vi "2DScan.vi"() -> ()   [LabVIEW 2014]
uses:
  <vilib>/vision/driver/IMAQdx.llb/IMAQdx Acquisition Mode.ctl
  <vilib>/vision/driver/IMAQdx.llb/IMAQdx Buffer Number Mode.ctl
  <vilib>/vision/driver/NI_Vision_Acquisition_Software.lvlib
panel:
  in  "Distance(V)":dbl
  in  "Boolean":bool
  out "RealPositionX":dbl
  out "Processed Frames/s":dbl
  in  "Step(V) Y":dbl=0.1
  out "RealPositionY":dbl
  in  "Step(V) X":dbl=0.1
  in  "pfVoltage in 2":sgl
  in  "pfVoltage in":sgl
  in  "Camera Name":refnum<k21>="cam0" caption="IMAQdx Session"
  in  "Stop":bool
  out "Image":T1(plugin-control)
  out "Buffer Number":u32
  out "error out":errorcluster
  in  "MG17Piezo X":refnum<k7>(container)
  in  "MG17Piezo Y":refnum<k7>(container)
  in  "MG17Piezo Z":refnum<k7>(container)
  # "2DScan"
  # "Randomic"
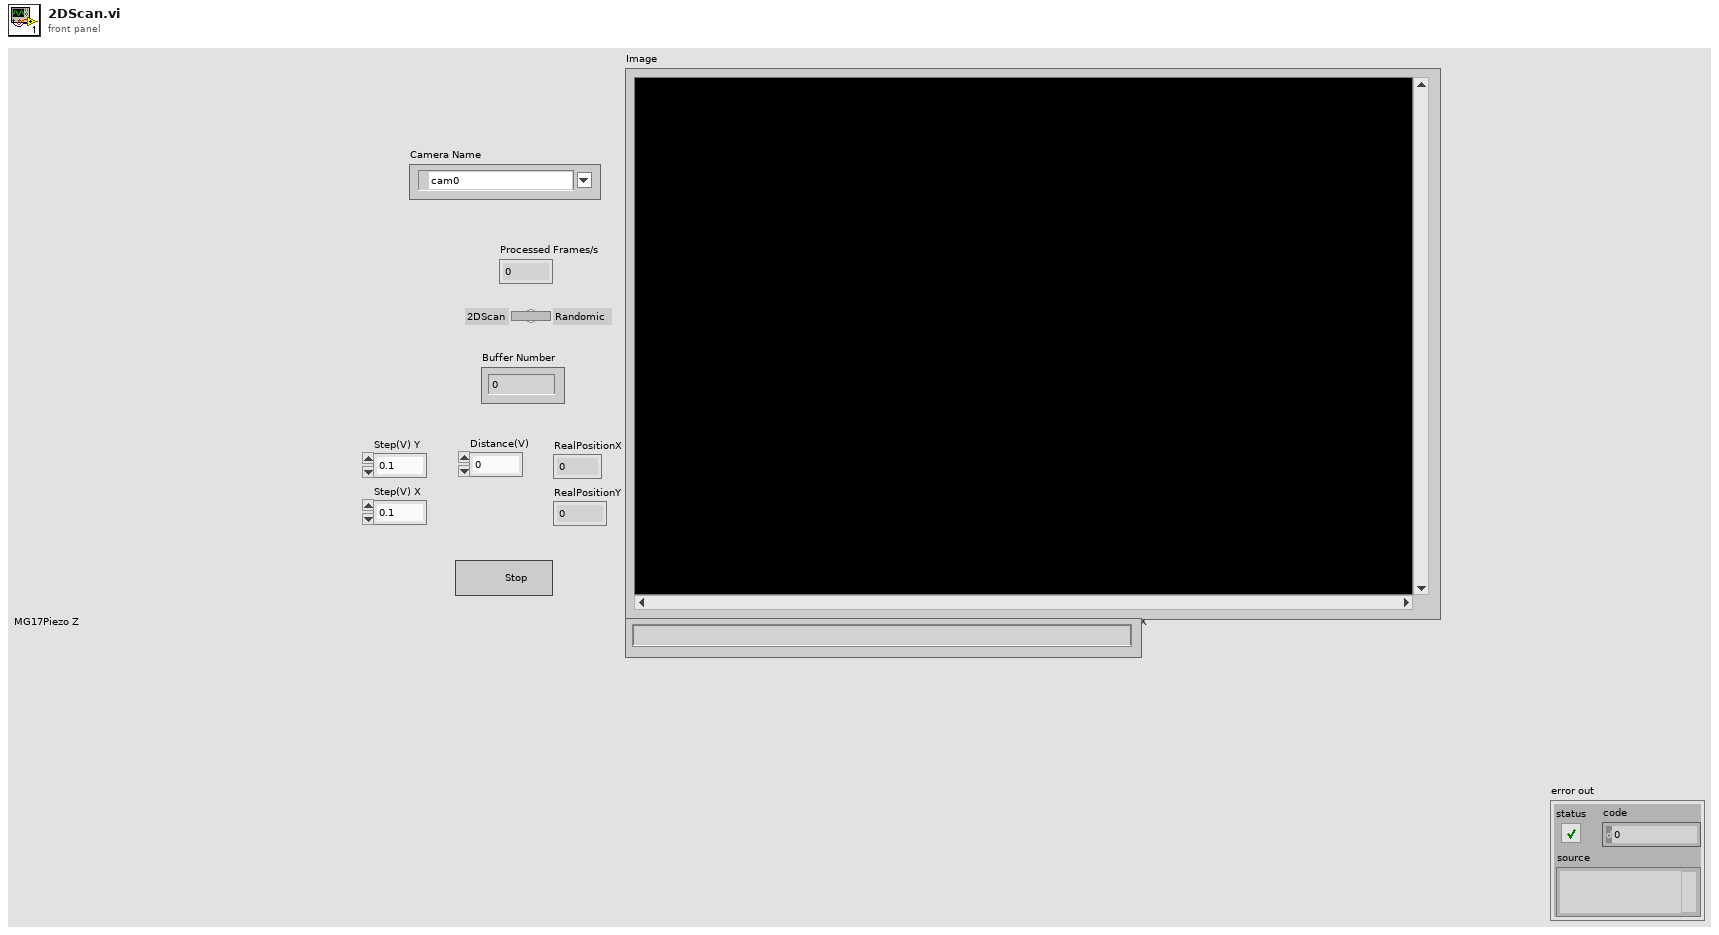
[diagram p1: front panel]
types:
  T1 = typedef "IMAQ Image.ctl" = refnum<image>
  T2 = typedef "NI_Vision_Acquisition_Software.lvlib/IMAQdx Acquisition Mode.ctl" = enum32{"One Shot", "Continuous"}
  T3 = typedef "IMAQdx.ctl" = refnum<k21>
  T4 = typedef "NI_Vision_Acquisition_Software.lvlib/IMAQdx Buffer Number Mode.ctl" = enum32{"Next", "Last", "Buffer Number"}
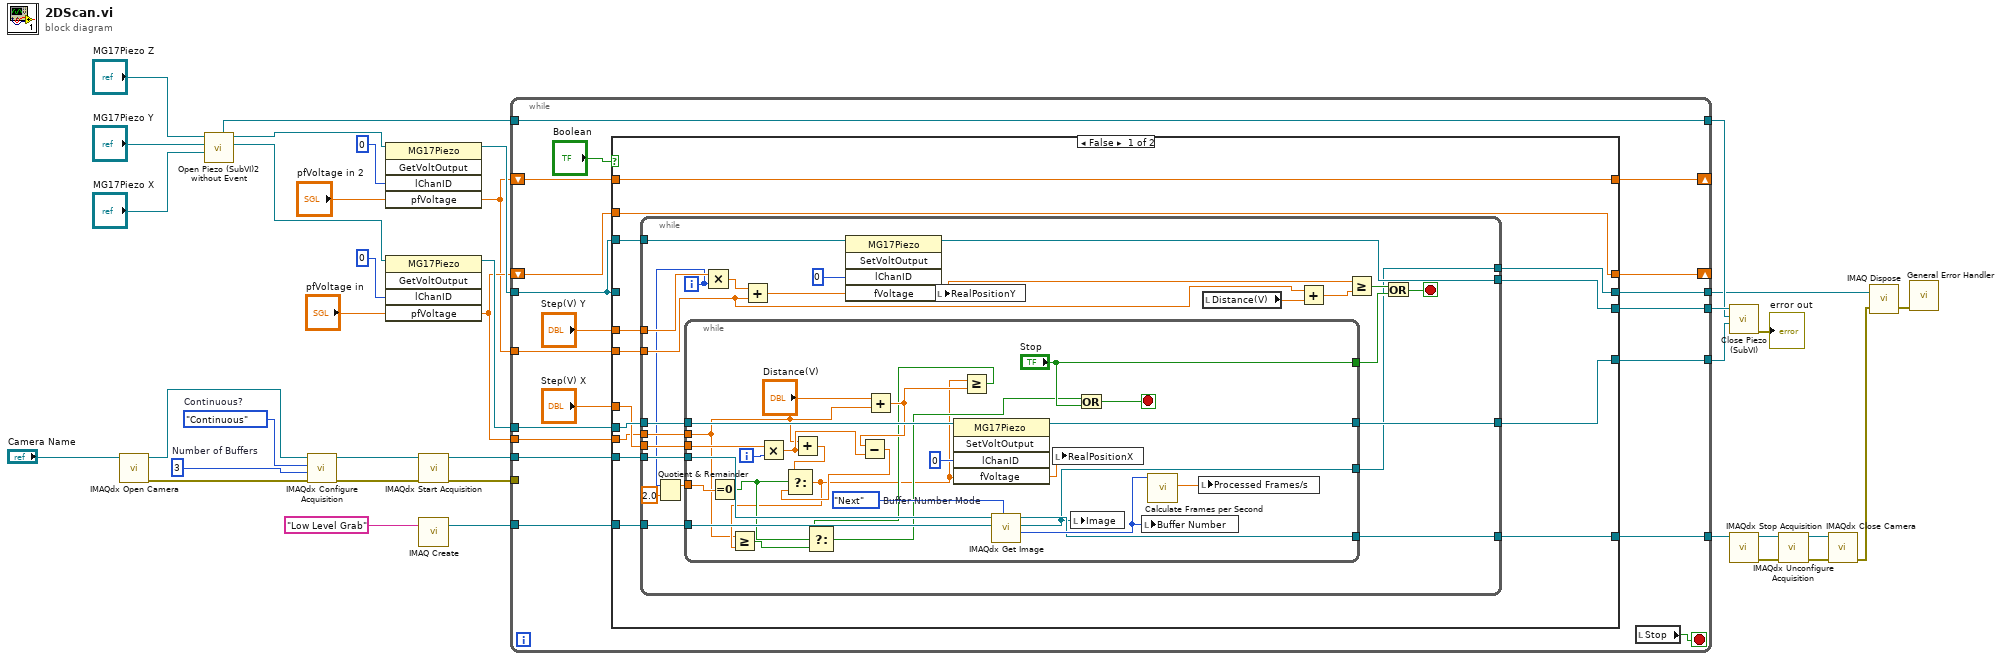
[diagram p0: block diagram]
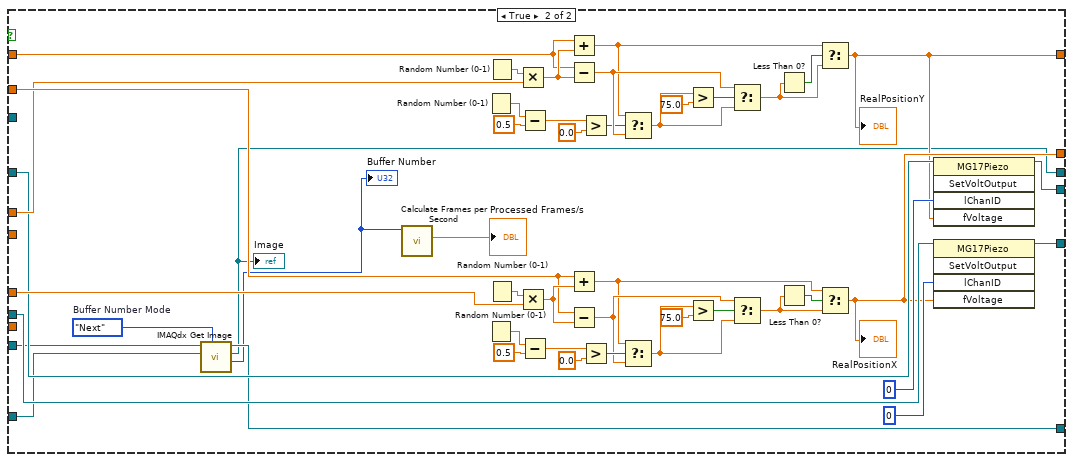
[diagram p2: hidden frame]
diagram:
  w26 = u32 3  # Number of Buffers
  w27 = IMAQdx_Acquisition_Mode."Continuous"  # Continuous?
  n1 = call <vilib>:"IMAQdx Open Camera.vi"("Session In"="Camera Name") -> ("error out"=w17:errorcluster, "Session Out"=w18:T3)  [unwired: 2 in, 7 out]
  n2 = call "Open Piezo (SubVI)2 without Event.vi"("MG17Piezo X"="MG17Piezo X", "MG17Piezo Y"="MG17Piezo Y", "MG17Piezo Z"="MG17Piezo Z") -> ("MG17 X"=w14:refnum<k7>, "MG17 Y"=w11:refnum<k7>, "MG17 Z"=w8:refnum<k7>)  [unwired: 3 in, 3 out]
  n3 = call <vilib>:"IMAQdx Configure Acquisition.vi"("error in"=w17, "Number of Buffers"=w26, "Continuous?"=w27, "Session In"=w18) -> ("error out"=w29:errorcluster, "Session Out"=w31:T3)  [unwired: 6 out]
  n4 = invoke class="MG17Piezo" method="GetVoltOutput"(reference=w11, "lChanID"=0, "pfVoltage"="pfVoltage in 2") -> (reference out=w9:refnum<k7>, "pfVoltage"=w3:sgl)  [unwired: 2 in, 3 out]
  n5 = invoke class="MG17Piezo" method="GetVoltOutput"(reference=w14, "lChanID"=0, "pfVoltage"="pfVoltage in") -> (reference out=w10:refnum<k7>, "pfVoltage"=w4:sgl)  [unwired: 2 in, 3 out]
  n6 = call <vilib>:"IMAQdx Start Acquisition.vi"("error in"=w29, "Session In"=w31) -> ("error out"=w28:errorcluster, "Session Out"=w30:T3)  [unwired: 8 out]
  n7 = call "IMAQ Create"("Image Name"="Low Level Grab") -> ("New Image"=w33:T1)  [unwired: 3 in, 2 out]
  n8 = while {
    tunnel: [w39] -> w2
    tunnel: w28 -> [_]
    tunnel: w30 -> [w42]
    tunnel: w33 -> [w41]
    tunnel: w10 -> [w50]
    tunnel: w9 -> [w48]
    tunnel: w8 -> [w56]
    shift-right: [w47] -> _
    shift-left: w4 -> [w54]
    shift-right: [w46] -> _
    shift-left: w3 -> [w51]
    tunnel: [w44] -> w7
    tunnel: [w45] -> w6
    tunnel: [w56] -> w5
    tunnel: w4 -> [w49]
    tunnel: w3 -> [w43]
    tunnel: [w38] -> w1
    stop <- w40 stop-if-true
    n9 = case shown="False" "Boolean" {
      tunnel: "Step(V) X" -> [w68 w154]
      tunnel: w54 -> [w62 w153]
      tunnel: "Step(V) Y" -> [w67 w138]
      tunnel: w51 -> [w61 w137]
      tunnel: w50 -> [w70 w135]
      tunnel: w48 -> [w69 _]
      tunnel: w49 -> [w66 _]
      tunnel: w48 -> [_ w133]
      tunnel: [w62 w132] -> w47
      tunnel: [w61 w131] -> w46
      tunnel: [w64 w130] -> w45
      tunnel: [w63 w129] -> w44
      tunnel: w43 -> [w65 _]
      tunnel: [w60 w126] -> w39
      tunnel: w42 -> [w59 w124]
      tunnel: w41 -> [w58 w123]
      tunnel: [w57 w122] -> w38
      frame False {
        n10 = while {
          tunnel: w66 -> [w94]
          tunnel: w70 -> [w93]
          tunnel: w65 -> [w81]
          tunnel: w69 -> [w87]
          tunnel: w68 -> [w86]
          tunnel: w67 -> [w83]
          tunnel: [w85] -> w64
          tunnel: [w84] -> w63
          tunnel: [w77] -> w60
          tunnel: w59 -> [w76]
          tunnel: w58 -> [w75]
          tunnel: [w74] -> w57
          i -> [w73]
          stop <- w90 stop-if-true
          n11 = Quotient & Remainder(x=w73, y=sgl 2.0) -> (x-y*floor(x/y)=w71:sgl)  [unwired: 1 out]
          n12 = while {
            tunnel: w94 -> [w95]
            tunnel: w93 -> [w118]
            tunnel: w86 -> [w115]
            tunnel: [w117] -> w85
            tunnel: ["Stop"] -> w79
            tunnel: [w109] -> w77
            tunnel: w76 -> [w108]
            tunnel: w75 -> [w107]
            tunnel: [w106] -> w74
            tunnel: w71 -> [w105]
            i -> [w116]
            stop <- w121 stop-if-true
            w112 = IMAQdx_Buffer_Number_Mode."Next"  # Buffer Number Mode
            n13 = Equal To 0?(x=w105) -> (x = 0?=w100:bool)
            n14 = Multiply(x=w115, y=w116) -> (x*y=w102:dbl)
            n15 = Add(x=w95, y=w102) -> (x+y=w104:dbl)
            n16 = Add(x="Distance(V)", y=w95) -> (x+y=w103:dbl)
            n17 = Subtract(x=w103, y=w102) -> (x-y=w101:dbl)
            n18 = Select(t=w104, s=w100, f=w101) -> (s? t:f=w96:dbl)
            n19 = Greater Or Equal?(x=w95, y=w96) -> (x >= y?=w97:bool)
            n20 = invoke class="MG17Piezo" method="SetVoltOutput"(reference=w118, "lChanID"=0, "fVoltage"=w96) -> (reference out=w117:refnum<k7>, "fVoltage"=w113:sgl)  [unwired: 2 in, 3 out]
            n21 = Greater Or Equal?(x=w96, y=w103) -> (x >= y?=w98:bool)
            n22 = Select(t=w98, s=w100, f=w97) -> (s? t:f=w99:bool)
            n23 = call <vilib>:"IMAQdx Get Image.vi"("Buffer Number Mode (Next)"=w112, "Image In"=w107, "Session In"=w108) -> ("Buffer Number Out"=w111:u32, "Image Out"=w106:T1, "Session Out"=w109:T3)  [unwired: 2 in, 4 out]
            n24 = local write "RealPositionX"(w113) -> ()
            n25 = local write "Image"(w106) -> ()
            n26 = Or(x=w99, y="Stop") -> (x .or. y?=w121:bool)
            n27 = local write "Buffer Number"(w111) -> ()
            n28 = call <vilib>:"Calculate Frames per Second.vi"("Buffer Number"=w111) -> ("Processed Frames/s"=w110:dbl)  [unwired: 8 in, 2 out]
            n29 = local write "Processed Frames/s"(w110) -> ()
          }
          n30 = Multiply(x=w83, y=w73) -> (x*y=w82:dbl)
          n31 = Add(x=w82, y=w81) -> (x+y=w80:dbl)
          n32 = invoke class="MG17Piezo" method="SetVoltOutput"(reference=w87, "lChanID"=0, "fVoltage"=w80) -> (reference out=w84:refnum<k7>, "fVoltage"=w78:sgl)  [unwired: 2 in, 3 out]
          n33 = local write "RealPositionY"(w78) -> ()
          n34 = local read "Distance(V)"() -> (w89:dbl)
          n35 = Add(x=w81, y=w89) -> (x+y=w91:dbl)
          n36 = Greater Or Equal?(x=w78, y=w91) -> (x >= y?=w92:bool)
          n37 = Or(x=w92, y=w79) -> (x .or. y?=w90:bool)
        }
      }
      frame True {
        w127 = IMAQdx_Buffer_Number_Mode."Next"  # Buffer Number Mode
        n38 = call <vilib>:"IMAQdx Get Image.vi"("Buffer Number Mode (Next)"=w127, "Image In"=w123, "Session In"=w124) -> ("Buffer Number Out"=w125:u32, "Image Out"=w122:T1, "Session Out"=w126:T3)  [unwired: 2 in, 4 out]
        "Image" <- w122
        "Buffer Number" <- w125
        n39 = call <vilib>:"Calculate Frames per Second.vi"("Buffer Number"=w125) -> ("Processed Frames/s"=→"Processed Frames/s":dbl)  [unwired: 8 in, 2 out]
        n40 = Random Number (0-1)() -> (number: 0 to 1=w147:dbl)
        n41 = Random Number (0-1)() -> (number: 0 to 1=w161:dbl)
        n42 = Random Number (0-1)() -> (number: 0 to 1=w142:dbl)
        n43 = Random Number (0-1)() -> (number: 0 to 1=w166:dbl)
        n44 = Multiply(x=w142, y=w138) -> (x*y=w143:dbl)
        n45 = Multiply(x=w166, y=w154) -> (x*y=w165:dbl)
        n46 = Subtract(x=w147, y=0.5) -> (x-y=w148:dbl)
        n47 = Subtract(x=w161, y=0.5) -> (x-y=w160:dbl)
        n48 = Add(x=w137, y=w143) -> (x+y=w139:dbl)
        n49 = Subtract(x=w137, y=w143) -> (x-y=w151:dbl)
        n50 = Add(x=w153, y=w165) -> (x+y=w156:dbl)
        n51 = Subtract(x=w153, y=w165) -> (x-y=w157:dbl)
        n52 = Greater?(x=w148, y=0.0) -> (0:w150:bool)
        n53 = Greater?(x=w160, y=0.0) -> (0:w158:bool)
        n54 = Select(t=w139, s=w150, f=w151) -> (s? t:f=w152:dbl)
        n55 = Select(t=w156, s=w158, f=w157) -> (s? t:f=w155:dbl)
        n56 = Greater?(x=w152, y=75.0) -> (0:w140:bool)
        n57 = Greater?(x=w155, y=75.0) -> (0:w168:bool)
        n58 = Select(t=w151, s=w140, f=w152) -> (s? t:f=w145:dbl)
        n59 = Select(t=w157, s=w168, f=w155) -> (s? t:f=w163:dbl)
        n60 = Less Than 0?(x=w145) -> (x < 0?=w144:bool)
        n61 = Less Than 0?(x=w163) -> (x < 0?=w164:bool)
        n62 = Select(t=w139, s=w144, f=w145) -> (s? t:f=w131:dbl)
        "RealPositionY" <- w131
        n63 = Select(t=w156, s=w164, f=w163) -> (s? t:f=w132:dbl)
        "RealPositionX" <- w132
        n64 = invoke class="MG17Piezo" method="SetVoltOutput"(reference=w133, "lChanID"=0, "fVoltage"=w131) -> (reference out=w129:refnum<k7>)  [unwired: 2 in, 4 out]
        n65 = invoke class="MG17Piezo" method="SetVoltOutput"(reference=w135, "lChanID"=0, "fVoltage"=w132) -> (reference out=w130:refnum<k7>)  [unwired: 2 in, 4 out]
      }
    }
    n66 = local read "Stop"() -> (w40:bool)
  }
  n67 = call "Close Piezo (SubVI).vi"("MG17 X"=w6, "MG17 Z"=w5, "MG17 Y"=w7) -> ("error out"=→"error out":errorcluster)  [unwired: 8 in]
  n68 = call <vilib>:"IMAQdx Stop Acquisition.vi"("Session In"=w2) -> ("error out"=w22:errorcluster, "Session Out"=w23:T3)  [unwired: 1 in, 8 out]
  n69 = call <vilib>:"IMAQdx Unconfigure Acquisition.vi"("error in"=w22, "Session In"=w23) -> ("error out"=w25:errorcluster, "Session Out"=w24:T3)  [unwired: 8 out]
  n70 = call <vilib>:"IMAQdx Close Camera.vi"("error in"=w25, "Session In"=w24) -> ("error out"=w21:errorcluster)  [unwired: 9 out]
  n71 = call "IMAQ Dispose"("Image"=w1, "error in (no error)"=w21) -> ("error out"=w20:errorcluster)  [unwired: 4 in]
  n72 = call <vilib>:"General Error Handler.vi"("error in (no error)"=w20) -> ()  [unwired: 2 in, 13 out]
